vi "parse controls plan.vi"(8 "error in (no error)":errorcluster, 11 "plan in":string) -> (0 "error out":errorcluster, 3 "plan out":T1)   [LabVIEW 2024, in "controls manager.lvlib"]
uses:
  controls manager.lvlib
  controls plan.ctl
  key value pair.ctl
  section.ctl
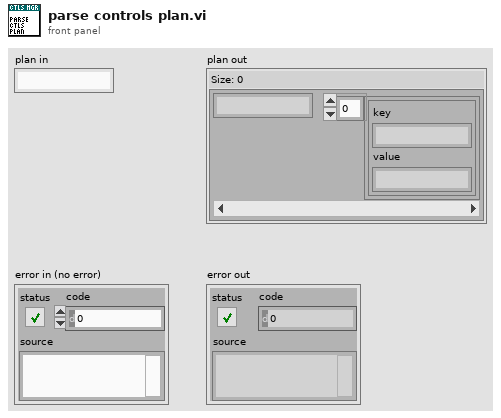
[diagram p1: front panel]
types:
  T1 = typedef "controls manager.lvlib/controls plan.ctl" = map{string, T2[]}
  T2 = typedef "controls manager.lvlib/key value pair.ctl" = cluster{"key":string, "value":string}
  T3 = typedef "controls manager.lvlib/section.ctl" = cluster{"section":string, "settings":T2[]}
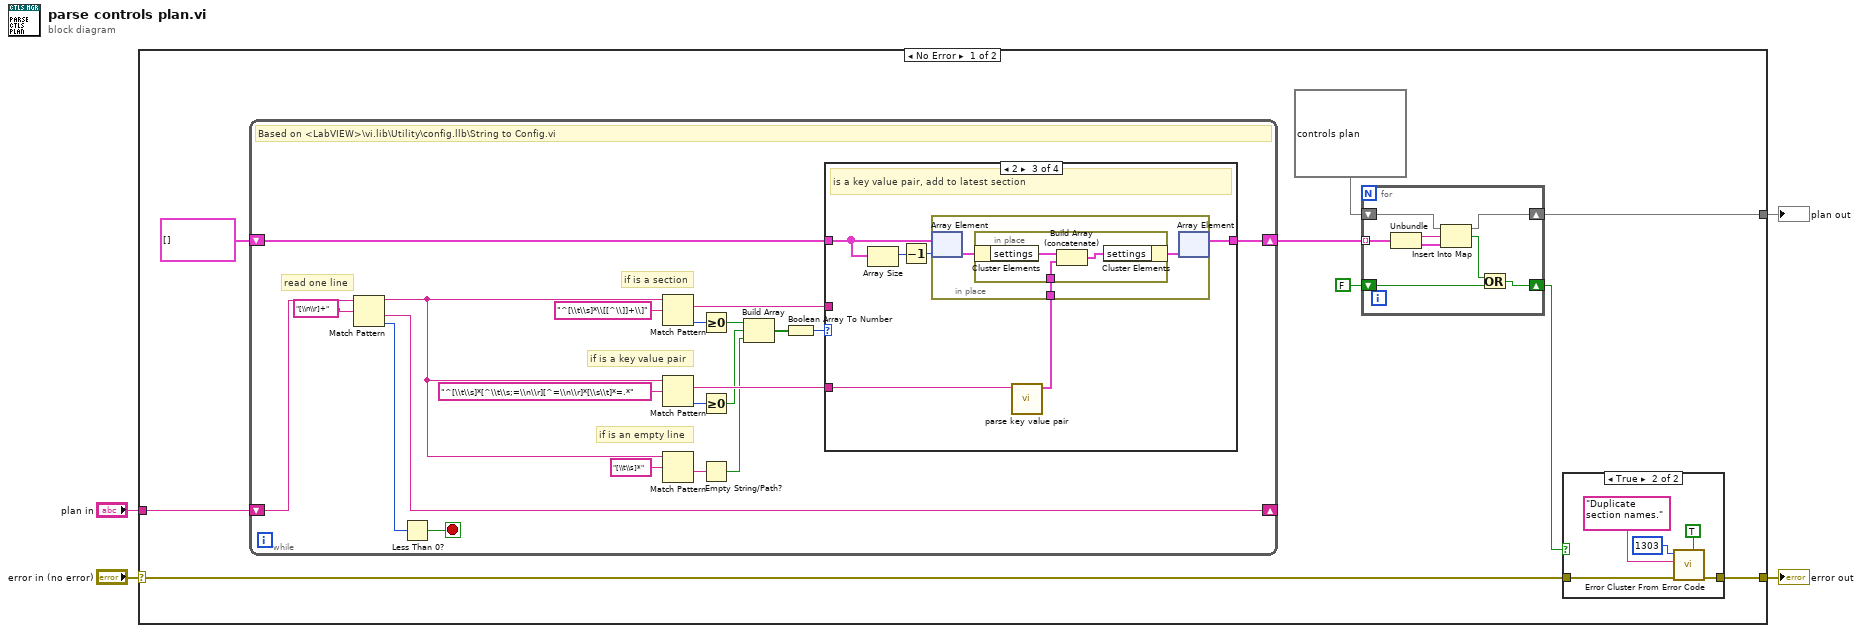
[diagram p0: block diagram]
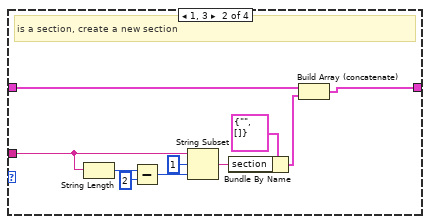
[diagram p4: hidden frame]
diagram:
  n1 = case shown="No Error" "error in (no error)" {
    selector: "error in (no error)" -> [w8 w73]
    tunnel: "plan in" -> [w12 _]
    tunnel: [w6 w73] -> w2
    tunnel: [w5 _] -> w1
    frame No Error {
      n2 = while {
        shift-right: [w22] -> w11
        shift-left: T3[] [] ("sections") -> [w33]
        shift-right: [w28] -> _
        shift-left: w12 -> [w23]
        stop <- w30 stop-if-true
        # "if is an empty line"
        # "if is a key value pair"
        # "if is a section"
        # "read one line"
        # "Based on <LabVIEW>\\vi.lib\\Utility\\config.llb\\String to Config.vi"
        n3 = Match Pattern(string=w23, regular expression="[\\n\\r]+") -> (before substring=w26:string, after substring=w28:string, offset past match=w29:i32)  [unwired: 1 in, 1 out]
        n4 = Less Than 0?(x=w29) -> (x < 0?=w30:bool)
        n5 = Match Pattern(string=w26, regular expression="^[\\t\\s]*\\[[^\\]]+\\]") -> (match substring=w34:string, offset past match=w39:i32)  [unwired: 1 in, 2 out]
        n6 = Match Pattern(string=w26, regular expression="^[\\t\\s]*[^\\t\\s;=\\n\\r][^=\\n\\r]*[\\s\\t]*=.*") -> (match substring=w40:string, offset past match=w24:i32)  [unwired: 1 in, 2 out]
        n7 = Match Pattern(string=w26, regular expression="[\\t\\s]*") -> (after substring=w31:string)  [unwired: 1 in, 3 out]
        n8 = Greater Or Equal To 0?(x=w39) -> (x >= 0?=w38:bool)
        n9 = Greater Or Equal To 0?(x=w24) -> (x >= 0?=w37:bool)
        n10 = Empty String/Path?(string/path=w31) -> (empty?=w32:bool)
        n11 = Build Array(w38, w37, w32) -> (w36:bool[])
        n12 = Boolean Array To Number(Boolean array=w36) -> (number=w35:u32)
        n13 = case shown="2" w35 {
          tunnel: w34 -> [_ w44 _ _]
          tunnel: w40 -> [_ _ w54 _]
          tunnel: w33 -> [w41 w46 w57 w64]
          tunnel: [w41 w45 w52 w64] -> w22
          frame Default {
            # "it is a comment, skip it"
          }
          frame 1, 3 {
            # "is a section, create a new section"
            n14 = String Length(string=w44) -> (length=w49:i32)
            n15 = Subtract(x=w49, y=2) -> (x-y=w50:i32)
            n16 = String Subset(string=w44, offset (0)=1, length (rest)=w50) -> (substring=w47:string)
            n17 = Bundle By Name(cluster=T3 {"section"="", "settings"=[]} ("section"), "section"=w47) -> (w42:T3)
            n18 = Build Array (concatenate)(w46, w42) -> (w45:T3[])
          }
          frame 2 {
            # "is a key value pair, add to latest section"
            n19 = Array Size(array=w57) -> (size(s)=w55:i32)
            n20 = Decrement(x=w55) -> (x-1=w56:i32)
            n21 = call "parse key value pair.vi"("key value pair in"=w54) -> ("key value pair out"=w53:T2)  [unwired: 9 in, 1 out]
            n22 = in-place {
              in-place-border: w53 -> [w58]
              n23 = in-place-array #1(w57, w56) -> (w60:T3)
              n24 = in-place {
                in-place-border: w58 -> [w61]
                n25 = in-place-cluster #2(w60) -> ("settings"=w63:T2[])
                n26 = Build Array (concatenate)(w63, w61) -> (w62:T2[])
                n27 = in-place-cluster #2("settings"=w62) -> (w59:T3)
              }
              n28 = in-place-array #1(w59) -> (w52:T3[])  [unwired: 1 out]
            }
          }
          frame 4 {
            # "empty line"
          }
        }
      }
      n29 = for {
        tunnel: w11 -> [w72] mode=indexing
        shift-right: [w69] -> w5
        shift-left: T1 {} -> [w68]
        shift-right: [w65] -> w7
        shift-left: FALSE -> [w66]
        n30 = Unbundle(w72) -> ("section"=w71:string, "settings"=w70:T2[])
        n31 = Insert Into Map(map in=w68, key=w71, value=w70) -> (map out=w69:T1, key already included?=w67:bool)  [unwired: 1 out]
        n32 = Or(x=w67, y=w66) -> (x .or. y?=w65:bool)
      }
      n33 = case shown="True" w7 {
        tunnel: w8 -> [w14 w19]
        tunnel: [w14 w15] -> w6
        frame False {
        }
        frame True {
          n34 = call <vilib>:"Error Cluster From Error Code.vi"("is warning? (False)"=TRUE, "error in (no error)"=w19, "error message (\"\")"="Duplicate section names.", "error code (0)"=1303) -> ("error out"=w15:errorcluster)  [unwired: 5 in]
        }
      }
    }
    frame Error {
    }
  }
  "error out" <- w2
  "plan out" <- w1
